vi "ImageFile_GetSingleImage.vi"(8 "error in (no error)":errorcluster, 10 "File Path":path, 11 "Image In":T1) -> (0 "error out":errorcluster, 3 "New Image":T1)   [LabVIEW 2019]
uses:
  <vilib>/vision/Image Controls.llb/IMAQ Image.ctl
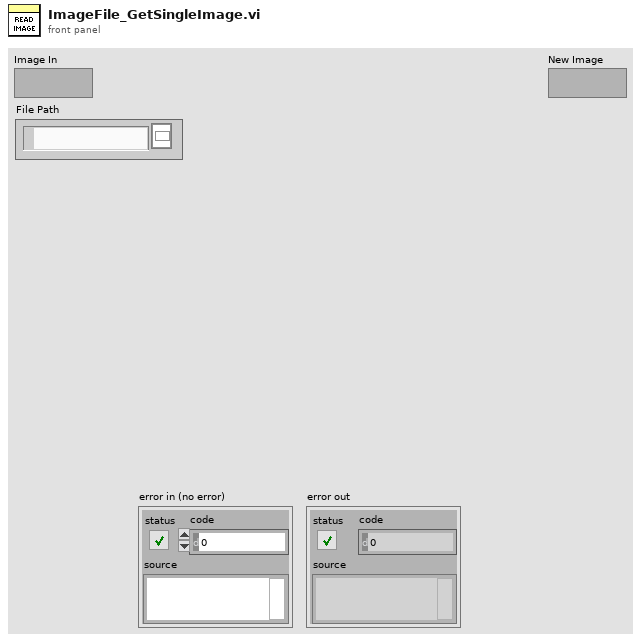
[diagram p1: front panel]
types:
  T1 = typedef "IMAQ Image.ctl" = refnum<image>
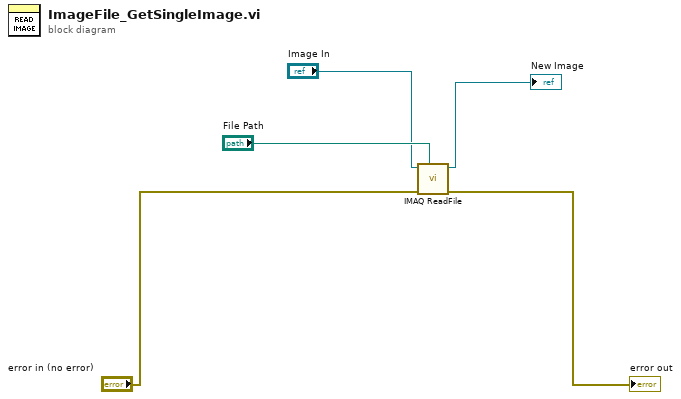
[diagram p0: block diagram]
diagram:
  n1 = call "IMAQ ReadFile"("File Path"="File Path", "error in (no error)"="error in (no error)", "Image"="Image In") -> ("error out"=→"error out":errorcluster, "Image Out"=→"New Image":T1)  [unwired: 4 in, 3 out]
